vi "clone.vi"(8 "error in (no error)":errorcluster, 11 "pCircle in":refnum<class "pCircle.lvclass">) -> (0 "error out":errorcluster, 3 "pCircle out":refnum<class "pCircle.lvclass">)   [LabVIEW 2017, in "pCircle.lvclass"]
uses:
  pCircle.lvclass
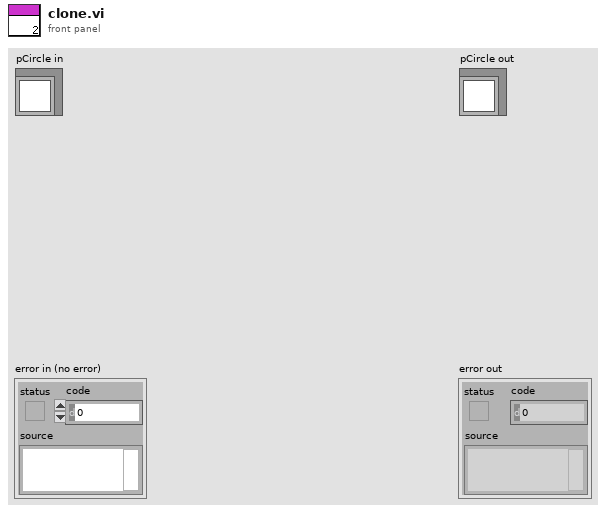
[diagram p1: front panel]
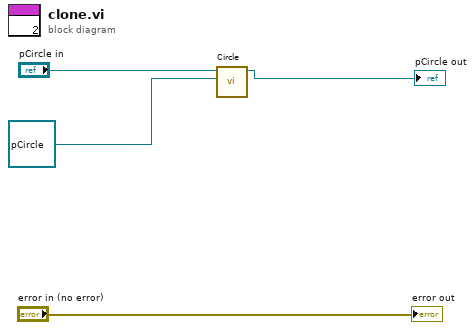
[diagram p0: block diagram]
diagram:
  n1 = call "Circle.vi"("target"=refnum<class "pCircle.lvclass"> refnum ("pCircle.lvclass"), "pCircle in"="pCircle in") -> ("pCircle out"=→"pCircle out":refnum<class "pCircle.lvclass">)  [unwired: 8 in, 1 out]
  "error out" <- "error in (no error)"
